vi "Act On Group.vi"(6 "Report Action":T1, 7 "Group Name":string, 8 "error in":errorcluster, 9 "Values":variant[](array[variant]), 10 "Parameters":string[](array[string]), 11 "TDMS in":refnum<class "TDMS.lvclass">) -> (0 "error out":errorcluster, 3 "TDMS out":refnum<class "TDMS.lvclass">)   [LabVIEW 2019, in "TDMS.lvlib" / "TDMS.lvclass"]
uses:
  TDMS.lvclass
  builds/Tools/Report.lvlibp/Custom Controls/Report Action.ctl
  TDMS.lvclass/TDMS.ctl
  builds/Tools/Report.lvlibp/Report.lvclass
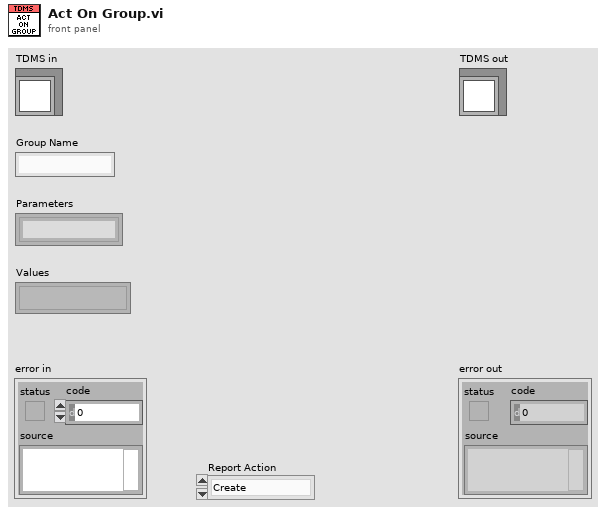
[diagram p1: front panel]
types:
  T1 = typedef "Report.lvlibp/Report.lvclass/Report Action.ctl" = enum16{"Create", "Append", "Destroy"}
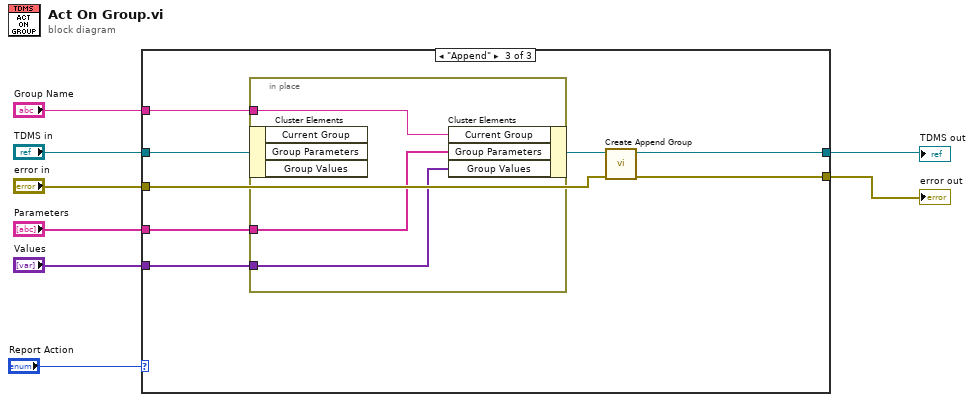
[diagram p0: block diagram]
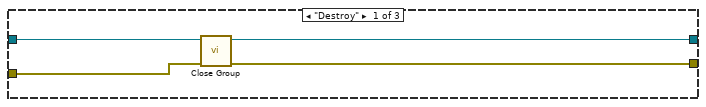
[diagram p2: hidden frame]
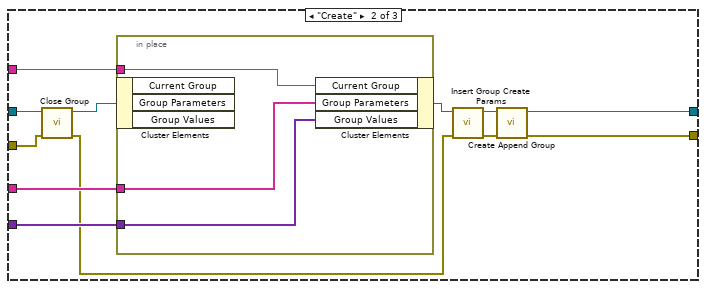
[diagram p3: hidden frame]
diagram:
  n1 = case shown="\"Append\"" "Report Action" {
    tunnel: "TDMS in" -> [w12 w16 w35]
    tunnel: "Group Name" -> [_ w24 w34]
    tunnel: "Parameters" -> [_ w23 w33]
    tunnel: "Values" -> [_ w22 w32]
    tunnel: "error in" -> [w11 w14 w29]
    tunnel: [w10 w21 w28] -> w2
    tunnel: [w9 w20 w30] -> w1
    frame "Destroy" {
      n2 = call "Close Group.vi"("error in"=w11, "TDMS in"=w12) -> ("error out"=w9:errorcluster, "TDMS out"=w10:refnum<class "TDMS.lvclass">)  [unwired: 8 in]
    }
    frame "Create" {
      n3 = call "Close Group.vi"("error in"=w14, "TDMS in"=w16) -> ("error out"=w13:errorcluster, "TDMS out"=w15:refnum<class "TDMS.lvclass">)  [unwired: 8 in]
      n4 = in-place {
        in-place-border: w24 -> [w25]
        in-place-border: w23 -> [w27]
        in-place-border: w22 -> [w26]
        n5 = in-place-cluster #1(w15) -> ()  [unwired: 3 out]
        n6 = in-place-cluster #1("Current Group"=w25, "Group Parameters"=w27, "Group Values"=w26) -> (w17:refnum<class "TDMS.lvclass">)
      }
      n7 = call "Insert Group Create Params.vi"("error in"=w13, "TDMS in"=w17) -> ("error out"=w19:errorcluster, "TDMS out"=w18:refnum<class "TDMS.lvclass">)  [unwired: 8 in]
      n8 = call "Create Append Group.vi"("error in"=w19, "TDMS in"=w18) -> ("error out"=w20:errorcluster, "TDMS out"=w21:refnum<class "TDMS.lvclass">)  [unwired: 8 in]
    }
    frame "Append" {
      n9 = in-place {
        in-place-border: w34 -> [w36]
        in-place-border: w33 -> [w38]
        in-place-border: w32 -> [w37]
        n10 = in-place-cluster #2(w35) -> ()  [unwired: 3 out]
        n11 = in-place-cluster #2("Current Group"=w36, "Group Parameters"=w38, "Group Values"=w37) -> (w31:refnum<class "TDMS.lvclass">)
      }
      n12 = call "Create Append Group.vi"("error in"=w29, "TDMS in"=w31) -> ("error out"=w30:errorcluster, "TDMS out"=w28:refnum<class "TDMS.lvclass">)  [unwired: 8 in]
    }
  }
  "error out" <- w1
  "TDMS out" <- w2
